vi "ACQ summary 1xtemp(add).vi"(3 "temp summary in":u32[][](array[numeric]), 4 "ChipID list":u16[](array[numeric]) format="%.0x", 5 "ACQtemp file path in":path caption="File path") -> (0 "temp summary out":u32[][](array[numeric]))   [LabVIEW 2015, in "VIPM2.lvlib"]
doc: "Totalitza events per chip i pixel d'una FPGA i d'un ACQtemp*"
uses:
  VIPM2.lvlib
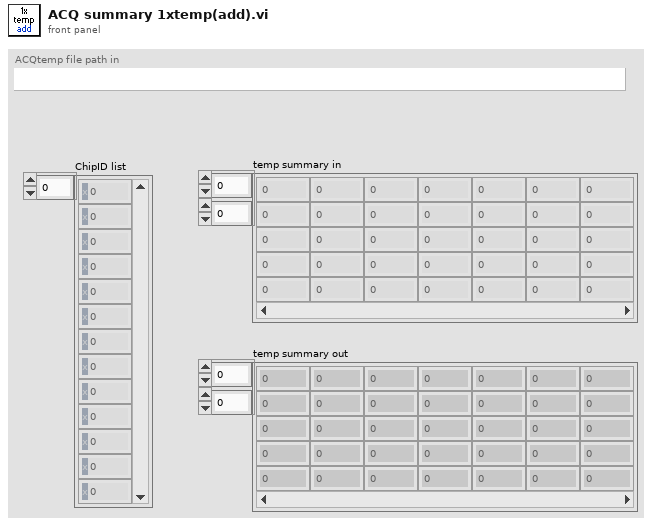
[diagram p1: front panel]
types:
  T1 = enum16{"big-endian, network order", "native, host order", "little-endian"}
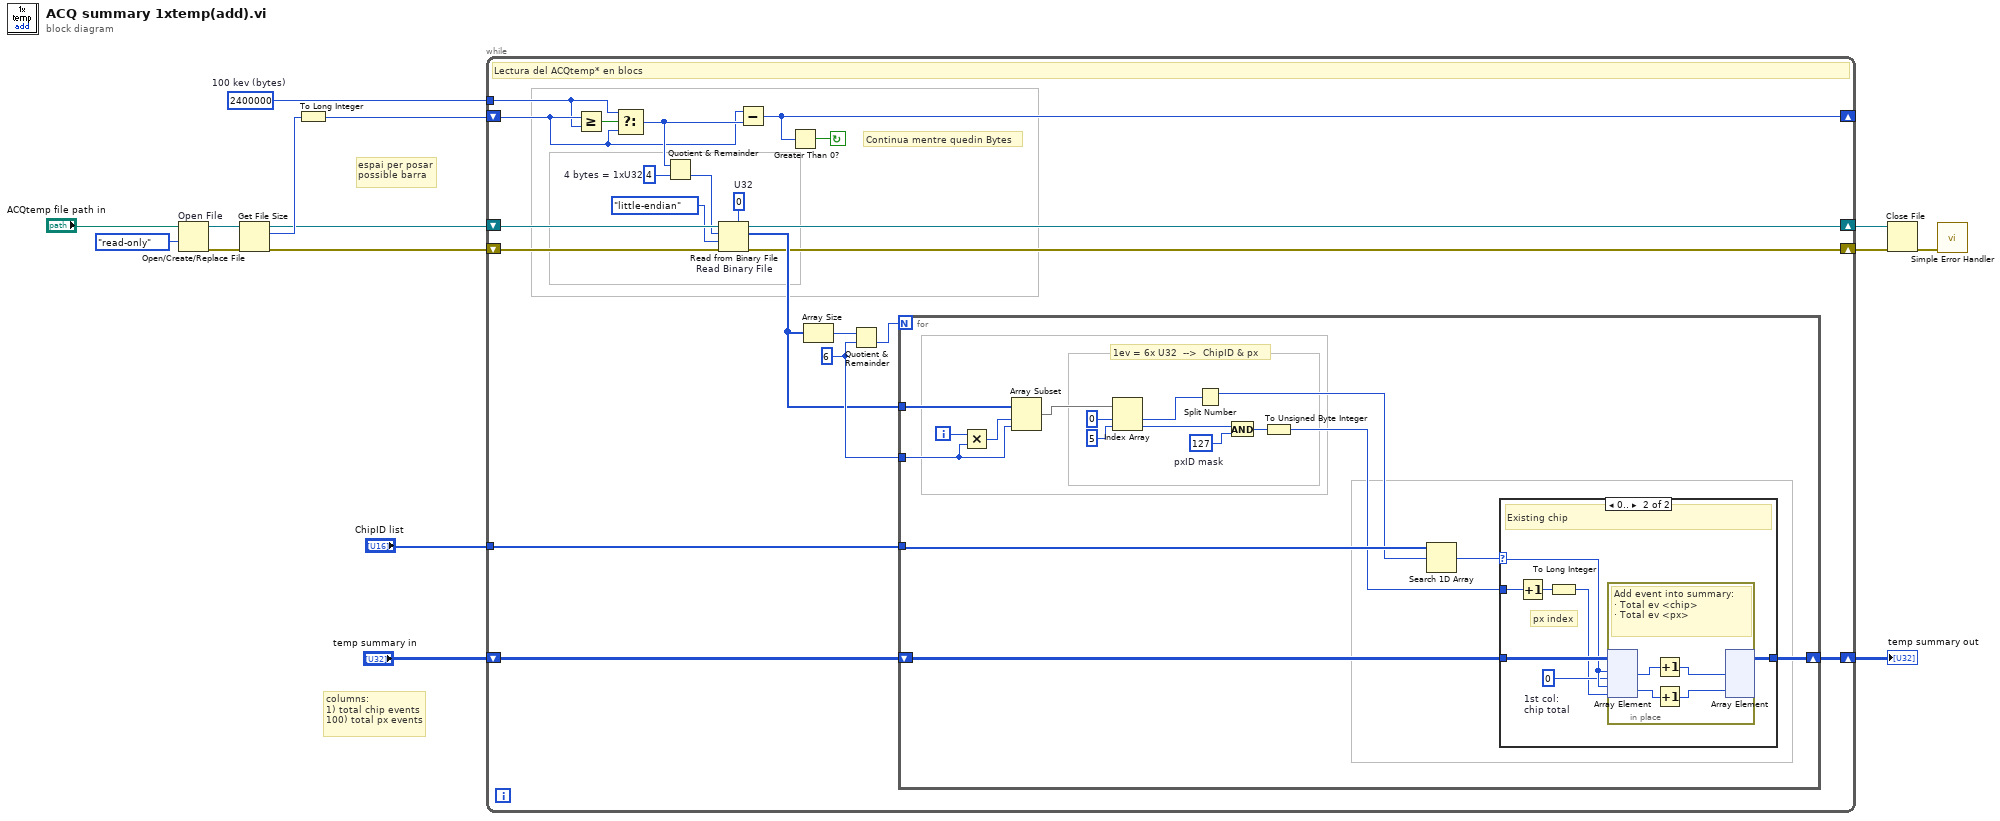
[diagram p0: block diagram]
diagram:
  w2 = 2400000  # 100 kev (bytes)
  # "columns:\n1) total chip events\n100) total px events"
  # "espai per posar\npossible barra"
  n1 = Open/Create/Replace File "Open File"(file path (use dialog)="ACQtemp file path in", access (0:read/write)=enum16{"read/write", "read-only", "write-only"}."read-only") -> (refnum out=w7:refnum<file>, error out=w6:errorcluster)  [unwired: 4 in, 1 out]
  n2 = Get File Size(file=w7, error in=w6) -> (refnum out=w5:refnum<file>, size (in bytes)=w8:i64, 0:w4:errorcluster)
  n3 = To Long Integer(number=w8) -> (32bit integer=w3:i32)
  n4 = while {
    tunnel: "ChipID list" -> [w29]
    shift-right: [w26] -> w12
    shift-left: w4 -> [w35]
    shift-right: [w25] -> w11
    shift-left: w5 -> [w34]
    shift-right: [w28] -> w13
    shift-left: "temp summary in" -> [w30]
    tunnel: w2 -> [w16]
    shift-right: [w19] -> _
    shift-left: w3 -> [w17]
    stop <- w20 continue-if-true
    w21 = 4  # 4 bytes = 1xU32
    w24 = u32 0  # U32
    w36 = 6 ("y")
    # "Continua mentre quedin Bytes"
    # "Lectura del ACQtemp* en blocs"
    n5 = Greater Or Equal?(x=w17, y=w16) -> (x >= y?=w23:bool)
    n6 = Select(t=w16, s=w23, f=w17) -> (s? t:f=w22:i32)
    n7 = Quotient & Remainder(x=w22, y=w21) -> (floor(x/y)=w18:i32)  [unwired: 1 out]
    n8 = Read from Binary File "Read Binary File"(5:w24, 8:w35, 9:T1."little-endian" ("byte order (0:big-endian, network order)"), 10:w18, 11:w34) -> (0:w26:errorcluster, 2:w33:u32[], 3:w25:refnum<file>)  [unwired: 1 in, 1 out]
    n9 = Subtract(x=w17, y=w22) -> (x-y=w19:i32)
    n10 = Greater Than 0?(x=w19) -> (x > 0?=w20:bool)
    n11 = Array Size(array=w33) -> (size(s)=w32:i32)
    n12 = Quotient & Remainder(x=w32, y=w36) -> (floor(x/y)=w31:i32)  [unwired: 1 out]
    n13 = for {
      N: w31 -> [_]
      tunnel: w33 -> [w47]
      tunnel: w36 -> [w43]
      shift-right: [w37] -> w28
      shift-left: w30 -> [w38]
      tunnel: w29 -> [w41]
      i -> [w45]
      w49 = u32 127  # pxID mask
      # "1ev = 6x U32  -->  ChipID & px"
      n14 = Multiply(x=w45, y=w43) -> (x*y=w44:i32)
      n15 = Array Subset "Array Subset"(array=w47, index=w44, length=w43) -> (w46:u32[])
      n16 = Index Array "Index Array"(array=w46, index #1=0 ("index"), index #2=5 ("index")) -> (element #1=w51:u32, element #2=w50:u32)
      n17 = Split Number(x=w51) -> (hi(x)=w40:u16)  [unwired: 1 out]
      n18 = And(x=w50, y=w49) -> (x .and. y?=w48:u32)
      n19 = To Unsigned Byte Integer(number=w48) -> (unsigned 8bit integer=w39:u8)
      n20 = Search 1D Array(1D array=w41, element=w40) -> (index of element=w42:i32)  [unwired: 1 in]
      n21 = case shown="0.." w42 {
        selector: w42 -> [_ w60]
        tunnel: w38 -> [w54 w61]
        tunnel: [w54 w55] -> w37
        tunnel: w39 -> [_ w59]
        frame -1, Default {
          # "Not existing chip"
        }
        frame 0.. {
          w58 = 0  # 1st col: chip total
          # "px index"
          # "Existing chip"
          n22 = Increment(x=w59) -> (x+1=w57:u8)
          n23 = To Long Integer(number=w57) -> (32bit integer=w56:i32)
          n24 = in-place "In Place Element Structure" {
            # "Add event into summary:\n· Total ev <chip>\n· Total ev <px>"
            n25 = in-place-array #1(w61, w60, w58, w60, w56) -> (w62:u32, w64:u32)
            n26 = Increment(x=w62) -> (x+1=w65:u32)
            n27 = Increment(x=w64) -> (x+1=w63:u32)
            n28 = in-place-array #1(w65, w63) -> (w55:u32[][])  [unwired: 4 out]
          }
        }
      }
    }
  }
  "temp summary out" <- w13
  n29 = Close File(refnum=w11, error in=w12) -> (error out=w10:errorcluster)  [unwired: 1 out]
  n30 = call <vilib>:"Simple Error Handler.vi"("error in (no error)"=w10) -> ()  [unwired: 4 in, 5 out]
